vi "LEDComms.vi"   [LabVIEW 2017]
uses:
  Implements/TypeDefs/IntakeState.ctl
  <vilib>/Rock Robotics/SystemInterfaces/i2clib/i2c_bus.ctl
  Global_Var-RefNum/LEDData.vi
types:
  T1 = typedef "ArmTargetPosition.ctl" = enum16{"Hold", "Switch", "Scale Low", "Scale High", "Climb", "Back Place"}
  T2 = typedef "WPI_DriverStationRobotMode2.ctl" = enum16{"Autonomous Disabled", "Autonomous Enabled", "Teleop Disabled", "Teleop Enabled", "Disconnected", "Finish", "Test Disabled", "Test Enabled", "Emergency Stopped"}
  T3 = typedef "IntakeState.ctl" = enum16{"Stop", "Forward", "Reverse", "Forward Open"}
  T4 = typedef "LEDAutoMode.ctl" = enum16{"Auto Line", "Auto Left Switch", "Auto Left Scale", "Auto Center Switch", "Auto Center Scale", "Auto Right Switch", "Auto Right Scale"}
  T5 = typedef "WPI_I2CDevRef.ctl" = cluster{"DevStatus":errorcluster, "Device Address":u8, "Handle":i32, "I2C Bus":T6}
  T6 = typedef "i2c_bus.ctl" = enum16{"I2C On-Board", "I2C MXP", "Invalid"}
  T7 = typedef "WPI_DriverStationAllianceInfo.ctl" = enum16{"Red", "Blue", "Invalid"}
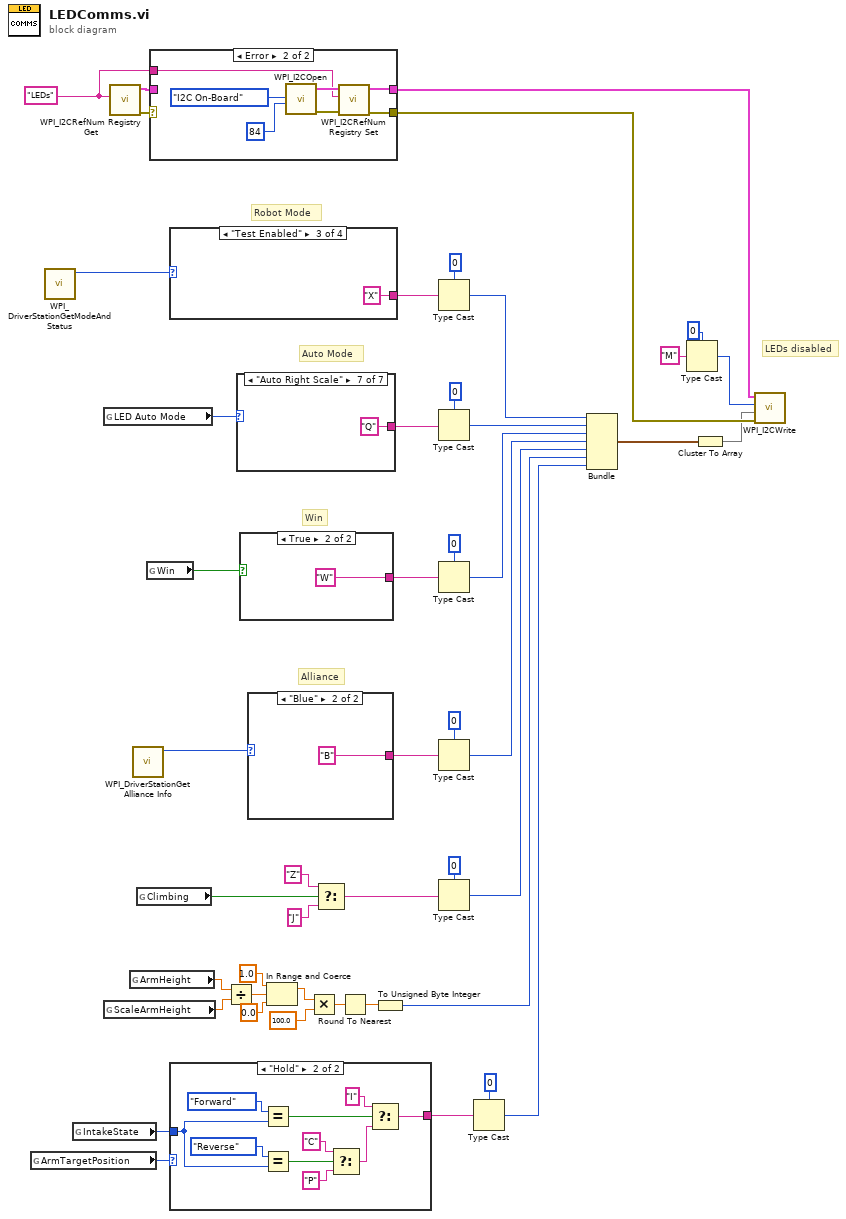
[diagram p0: block diagram]
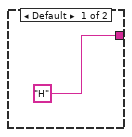
[diagram p2: hidden frame]
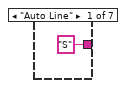
[diagram p4: hidden frame]
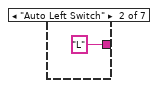
[diagram p5: hidden frame]
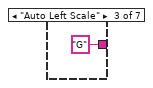
[diagram p6: hidden frame]
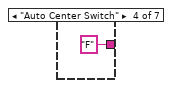
[diagram p7: hidden frame]
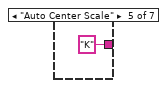
[diagram p8: hidden frame]
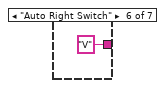
[diagram p9: hidden frame]
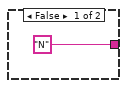
[diagram p10: hidden frame]
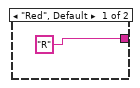
[diagram p11: hidden frame]
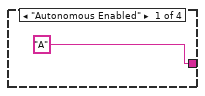
[diagram p12: hidden frame]
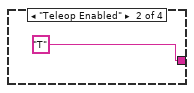
[diagram p13: hidden frame]
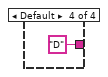
[diagram p14: hidden frame]
diagram:
  w22 = "LEDs" ("refnum name")
  # "LEDs disabled"
  # "Alliance"
  # "Win"
  # "Robot Mode"
  # "Auto Mode"
  n1 = global read "LEDData.vi" "ArmTargetPosition"() -> (w3:T1)
  n2 = call <vilib>:"WPI_DriverStationGetModeAndStatus.vi"() -> ("Robot Mode"=w29:T2)  [unwired: 10 in, 1 out]
  n3 = global read "LEDData.vi" "IntakeState"() -> (w1:T3)
  n4 = global read "LEDData.vi" "LED Auto Mode"() -> (w19:T4)
  n5 = global read "LEDData.vi" "ScaleArmHeight"() -> (w12:dbl)
  n6 = call <vilib>:"WPI_I2CRefNum Registry Get.vi"("refnum name"=w22) -> ("error out"=w20:errorcluster, "I2CDevRef"=w21:T5)  [unwired: 9 in]
  n7 = global read "LEDData.vi" "ArmHeight"() -> (w13:dbl)
  n8 = call <vilib>:"WPI_DriverStationGet Alliance Info.vi"() -> ("Alliance"=w38:T7)  [unwired: 6 in, 5 out]
  n9 = global read "LEDData.vi" "Climbing"() -> (w15:bool)
  n10 = global read "LEDData.vi" "Win"() -> (w18:bool)
  n11 = case shown="Error" w20 {
    selector: w20 -> [w49 _]
    tunnel: [w49 w51] -> w47
    tunnel: [w48 w52] -> w46
    tunnel: w21 -> [w48 _]
    tunnel: w22 -> [_ w50]
    frame No Error {
    }
    frame Error {
      n12 = call <vilib>:"WPI_I2COpen.vi"("Device Address"=u8 84, "I2C Bus"=i2c_bus."I2C On-Board") -> ("error out"=w54:errorcluster, "I2CDevRef"=w53:T5)  [unwired: 8 in]
      n13 = call <vilib>:"WPI_I2CRefNum Registry Set.vi"("error in (no error)"=w54, "refnum name"=w50, "I2CDevRef"=w53) -> ("error out"=w51:errorcluster, "I2CDevRef"=w52:T5)  [unwired: 7 in]
    }
  }
  n14 = case shown="\"Test Enabled\"" w29 {
    tunnel: ["A" "T" "X" "D"] -> w41
    frame "Autonomous Enabled" {
    }
    frame "Teleop Enabled" {
    }
    frame "Test Enabled" {
    }
    frame Default {
    }
  }
  n15 = case shown="\"Hold\"" w3 {
    tunnel: ["H" w62] -> w2
    tunnel: w1 -> [_ w69]
    frame Default {
    }
    frame "Hold" {
      n16 = Equal?(x=IntakeState."Forward", y=w69) -> (x = y?=w63:bool)
      n17 = Equal?(x=IntakeState."Reverse", y=w69) -> (x = y?=w67:bool)
      n18 = Select(t="C", s=w67, f="P") -> (s? t:f=w64:string)
      n19 = Select(t="I", s=w63, f=w64) -> (s? t:f=w62:string)
    }
  }
  n20 = Divide(x=w13, y=w12) -> (x/y=w11:dbl)
  n21 = case shown="\"Auto Right Scale\"" w19 {
    tunnel: ["S" "L" "G" "F" "K" "V" "Q"] -> w23
    frame "Auto Line" {
    }
    frame "Auto Left Switch" {
    }
    frame "Auto Left Scale" {
    }
    frame "Auto Center Switch" {
    }
    frame "Auto Center Scale" {
    }
    frame "Auto Right Switch" {
    }
    frame "Auto Right Scale" {
    }
  }
  n22 = case shown="True" w18 {
    tunnel: ["N" "W"] -> w31
    frame False {
    }
    frame True {
    }
  }
  n23 = case shown="\"Blue\"" w38 {
    tunnel: ["R" "B"] -> w36
    frame "Red", Default {
    }
    frame "Blue" {
    }
  }
  n24 = In Range and Coerce(upper limit=1.0, x=w11, lower limit=0.0) -> (coerced(x)=w8:dbl)  [unwired: 1 out]
  n25 = Multiply(x=w8, y=100.0) -> (x*y=w6:dbl)
  n26 = Select(t="Z", s=w15, f="J") -> (s? t:f=w14:string)
  n27 = Round To Nearest(number=w6) -> (nearest integer value=w5:dbl)
  n28 = To Unsigned Byte Integer(number=w5) -> (unsigned 8bit integer=w4:u8)
  n29 = Type Cast(type=u8 0, x=w41) -> (*(type *) &x=w40:u8)
  n30 = Type Cast(type=u8 0, x=w23) -> (*(type *) &x=w34:u8)
  n31 = Type Cast(type=u8 0, x=w31) -> (*(type *) &x=w32:u8)
  n32 = Type Cast(type=u8 0, x=w36) -> (*(type *) &x=w28:u8)
  n33 = Type Cast(type=u8 0, x=w14) -> (*(type *) &x=w26:u8)
  n34 = Type Cast(type=u8 0, x=w2) -> (*(type *) &x=w24:u8)
  n35 = Bundle(w40, w34, w32, w28, w26, w4, w24) -> (w30:cluster{u8, u8, u8, u8, u8, u8, u8})  [unwired: 1 in]
  n36 = Type Cast(type=u8 0, x="M") -> (*(type *) &x=w43:u8)
  n37 = Cluster To Array(cluster=w30) -> (array=w39:u8[])
  n38 = call <vilib>:"WPI_I2CWrite.vi"("error in (no error)"=w47, "I2CDataToSend"=w39, "I2CRegister"=w43, "I2CDevRef"=w46) -> ()  [unwired: 6 in, 2 out]
